vi "NewObjDlg.vi"(4 "error in (no error)":errorcluster, 5 "DevNo":i32, 6 "ObjName":string, 7 "Enable":bool=TRUE) -> (0 "error out":errorcluster, 1 "ObjLocation":string, 2 "OK":bool)   [LabVIEW 2010]
doc: "Displays a standard dialog box that prompts users to enter information, such as a user name and password.\n--------------------\n\nThis Express VI is configured as follows:\n\nMessage to Display to the User:Объект с заданными атрибутами в базе данных не найден. \nДля создания новой учётной записи введите адрес или описание объекта.\nThe inputs are: \nText Entry Box: ObjLocation"
panel:
  in  "ObjLocation":string
  out "String":string="Объект с заданными атрибутами в базе данных не найден. \nДля создания новой учётной записи введите адрес или описание объекта."
  in  "OK1":bool
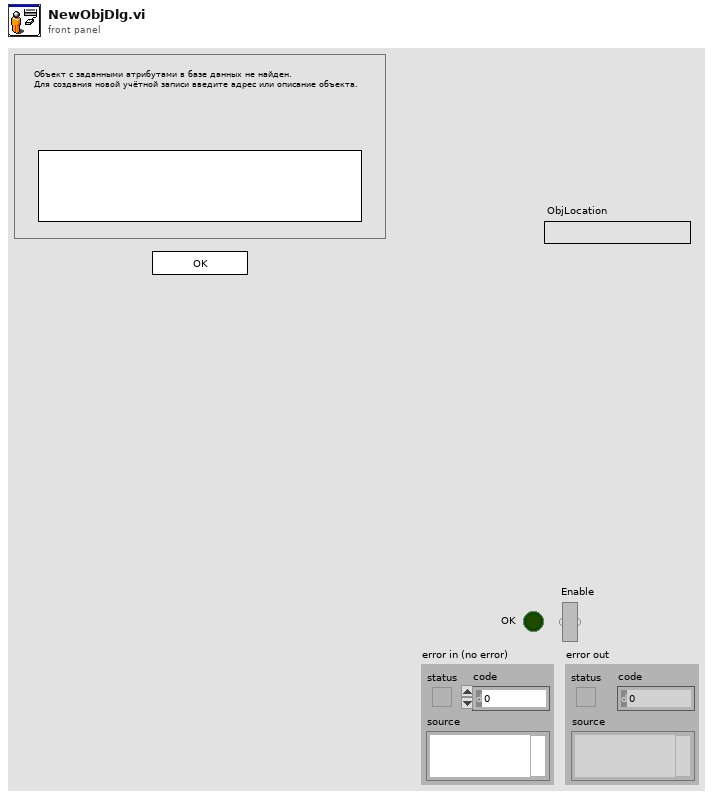
[diagram p1: front panel]
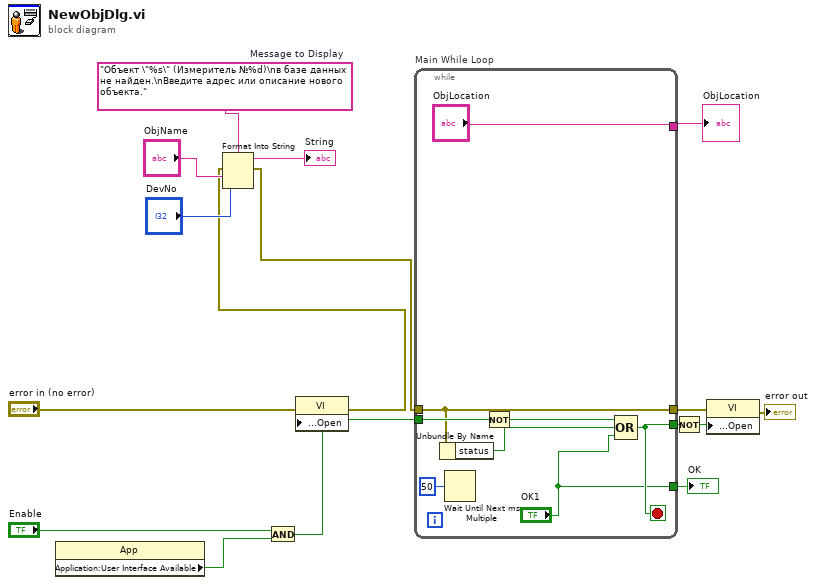
[diagram p0: block diagram]
diagram:
  w6 = "Объект \"%s\" (Измеритель №%d)\nв базе данных не найден.\nВведите адрес или описание нового объекта."  # Message to Display
  n1 = property class="App"() -> ("Application:User Interface Available"=w9:bool)  [unwired: 2 in, 2 out]
  n2 = And(x="Enable", y=w9) -> (x .and. y?=w10:bool)
  n3 = property class="VI"(error in="error in (no error)", "Front Panel Window:Open"=w10) -> (error out=w3:errorcluster)  [unwired: 1 in, 1 out]
  n4 = Format Into String(format string=w6, error in=w3, "ObjName", "DevNo") -> (resulting string=→"String":string, error out=w2:errorcluster)  [unwired: 1 in]
  n5 = while "Main While Loop" {
    tunnel: ["OK1"] -> w16
    tunnel: w10 -> [w23]
    tunnel: [w21] -> w14
    tunnel: w2 -> [w20]
    tunnel: [w20] -> w13
    tunnel: ["ObjLocation"] -> w8
    stop <- w21 stop-if-true
    n6 = Unbundle By Name(w20) -> ("status"=w19:bool)
    n7 = Wait Until Next ms Multiple(millisecond multiple=u32 50) -> ()  [unwired: 1 out]
    n8 = Not(x=w23) -> (.not. x?=w22:bool)
    n9 = Compound Arithmetic op=OR(w22, w19, "OK1") -> (w21:bool)
  }
  "OK" <- w16
  "ObjLocation" <- w8
  n10 = Not(x=w14) -> (.not. x?=w15:bool)
  n11 = property class="VI"(error in=w13, "Front Panel Window:Open"=w15) -> (error out=→"error out":errorcluster)  [unwired: 1 in, 1 out]
